vi "distance formula.vi"(10 "Point Y":dbl[](array[numeric]), 11 "Point X":dbl[](array[numeric])) -> (2 "Angle (rad)":dbl, 3 "Distance":dbl)   [LabVIEW 2018]
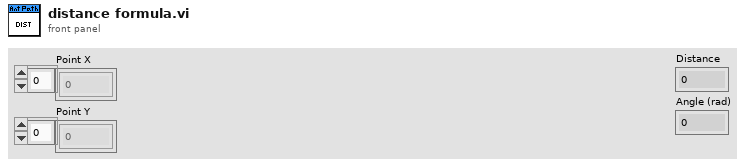
[diagram p1: front panel]
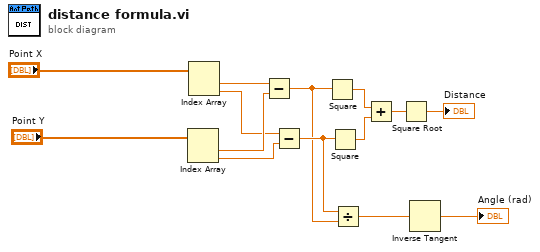
[diagram p0: block diagram]
diagram:
  n1 = Index Array(array="Point Y") -> (element #1=w13:dbl, element #2=w11:dbl)  [unwired: 2 in]
  n2 = Index Array(array="Point X") -> (element #1=w14:dbl, element #2=w12:dbl)  [unwired: 2 in]
  n3 = Subtract(x=w14, y=w13) -> (x-y=w3:dbl)
  n4 = Subtract(x=w12, y=w11) -> (x-y=w4:dbl)
  n5 = Square(x=w3) -> (x^2=w10:dbl)
  n6 = Square(x=w4) -> (x^2=w9:dbl)
  n7 = Divide(x=w4, y=w3) -> (x/y=w2:dbl)
  n8 = Add(x=w10, y=w9) -> (x+y=w8:dbl)
  n9 = Square Root(x=w8) -> (sqrt(x)=→"Distance":dbl)
  n10 = Inverse Tangent(1:w2) -> (0:→"Angle (rad)":dbl)
